vi "Set Temperature.vi"(5 "Air Temperature Setpoint (°C)":dbl=37.5 min=25.0 max=80.0 step=0.1, 11 "error in (no error)":errorcluster) -> (15 "error out":errorcluster)   [LabVIEW 2010]
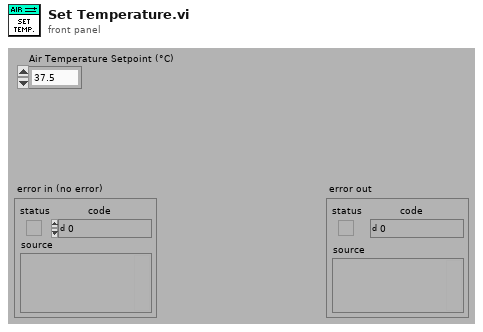
[diagram p1: front panel]
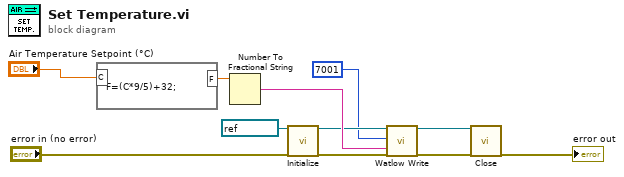
[diagram p0: block diagram]
diagram:
  n1 = formula code="F=(C*9/5)+32;"("C"="Air Temperature Setpoint (°C)") -> ("F"=w5:dbl)
  n2 = Number To Fractional String(number=w5) -> (F-format string=w4:string)  [unwired: 3 in]
  n3 = call <instrlib>:"Initialize.vi"("Comms Port"=refnum<visa-resource-name> "COM7", "Error In"="error in (no error)") -> ("UUT Port 2"=w3:refnum<visa-resource-name>, "Error Out"=w8:errorcluster)  [unwired: 16 out]
  n4 = call <instrlib>:"Watlow Write.vi"("PC Comms Port"=w3, "Parameter"=u32 7001, "Write Value"=w4, "Error In"=w8) -> ("Error Out"=w7:errorcluster)  [unwired: 15 in]
  n5 = call <instrlib>:"Close.vi"("PC Comms Port"=w3, "Error In"=w7) -> ("Error Out"=→"error out":errorcluster)  [unwired: 16 in, 1 out]
